vi "Error Dialog.vi"(0 "error":T1, 11 "error in (no error)":errorcluster) -> ()   [LabVIEW 2020]
uses:
  Error Description.ctl
panel:
  in  "OK":bool
  out "Details":string
  in  "Errors":string
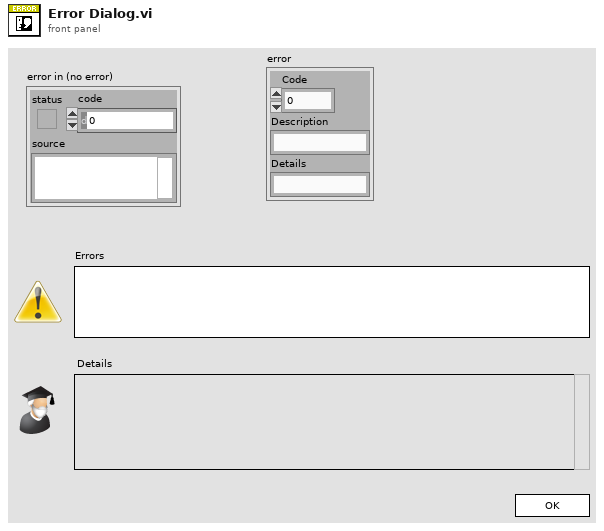
[diagram p1: front panel]
types:
  T1 = typedef "Error Description.ctl" = cluster{"Code":i32, "Description":string, "Details":string}
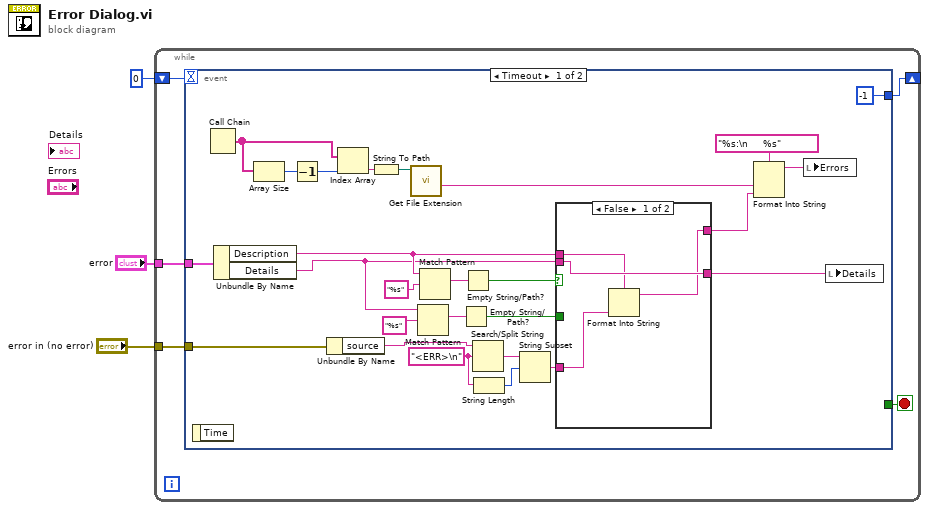
[diagram p0: block diagram]
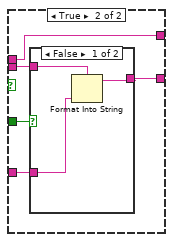
[diagram p2: hidden frame]
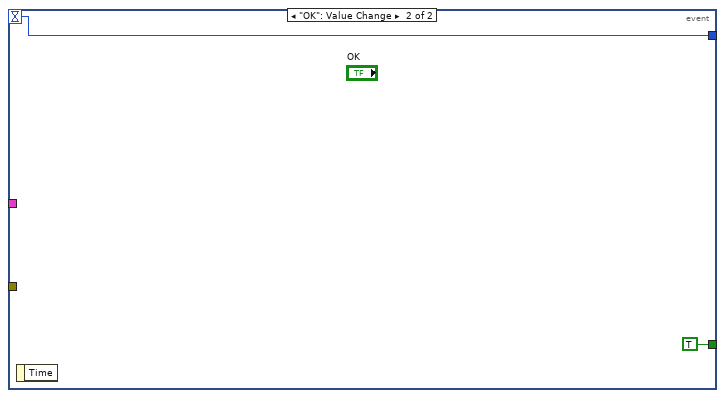
[diagram p4: hidden frame]
diagram:
  n1 = while {
    shift-right: [w7] -> _
    shift-left: 0 -> [w8]
    tunnel: "error in (no error)" -> [w5]
    tunnel: "error" -> [w4]
    stop <- w6 stop-if-true
    n2 = event shown="[0] Timeout" {
      selector: _ -> [_ _]
      dyn-events: _ -> [_ _]
      timeout: w8 -> [_ w49]
      tunnel: [-1 w49] -> w7
      tunnel: [_ TRUE] -> w6
      tunnel: w5 -> [w9 _]
      tunnel: w4 -> [w12 _]
      event Timeout {
        w18 = "<ERR>\n" ("search string/char (-)")
        n3 = event-data() -> ()  [unwired: 1 in, 1 out]
        n4 = Call Chain() -> (call chain=w31:string[])
        n5 = Unbundle By Name(w12) -> ("Description"=w11:string, "Details"=w10:string)
        n6 = Array Size(array=w31) -> (size(s)=w33:i32)
        n7 = Decrement(x=w33) -> (x-1=w32:i32)
        n8 = Unbundle By Name(w9) -> ("source"=w16:string)
        n9 = Index Array(array=w31, index=w32) -> (element=w30:string)
        n10 = String To Path(string=w30) -> (path=w29:path)
        n11 = call <vilib>:"Get File Extension.vi"("file"=w29) -> ("filename without extension"=w26:string)  [unwired: 6 in, 4 out]
        n12 = Match Pattern(string=w10, regular expression="%s") -> (match substring=w24:string)  [unwired: 1 in, 3 out]
        n13 = Match Pattern(string=w11, regular expression="%s") -> (match substring=w21:string)  [unwired: 1 in, 3 out]
        n14 = Empty String/Path?(string/path=w24) -> (empty?=w23:bool)
        n15 = Empty String/Path?(string/path=w21) -> (empty?=w15:bool)
        n16 = Search/Split String(string=w16, search string/char (-)=w18) -> (match + rest of string=w17:string)  [unwired: 1 in, 2 out]
        n17 = String Length(string=w18) -> (length=w19:i32)
        n18 = String Subset(string=w17, offset (0)=w19) -> (substring=w14:string)  [unwired: 1 in]
        n19 = case shown="False" w15 {
          tunnel: w23 -> [_ w43]
          tunnel: w10 -> [w38 w42]
          tunnel: [w38 w41] -> w22
          tunnel: w14 -> [w36 w40]
          tunnel: w11 -> [w37 w39]
          tunnel: [w35 w39] -> w13
          frame False {
            n20 = Format Into String(format string=w37, w36) -> (resulting string=w35:string)  [unwired: 2 in, 1 out]
          }
          frame True {
            n21 = case shown="False" w43 {
              tunnel: w42 -> [w46 w47]
              tunnel: [w45 w47] -> w41
              tunnel: w40 -> [w44 _]
              frame False {
                n22 = Format Into String(format string=w46, w44) -> (resulting string=w45:string)  [unwired: 2 in, 1 out]
              }
              frame True {
              }
            }
          }
        }
        n23 = Format Into String(format string="%s:\n     %s", w26, w13) -> (resulting string=w28:string)  [unwired: 2 in, 1 out]
        n24 = local write "Errors"(w28) -> ()
        n25 = local write "Details"(w22) -> ()
      }
      event "OK": Value Change {
        n26 = event-data() -> ()  [unwired: 1 in, 1 out]
      }
    }
  }
